vi "MyInterfaceMethod.vi"(0 "reference in":refnum<class "MyClass2.lvclass">, 1 "MyParameter":dbl, 5 "error in (no error)":errorcluster) -> (14 "reference out":refnum<class "MyClass2.lvclass">, 19 "error out":errorcluster)   [LabVIEW 2017, in "MyClass2.lvclass"]
uses:
  MyClass2.lvclass
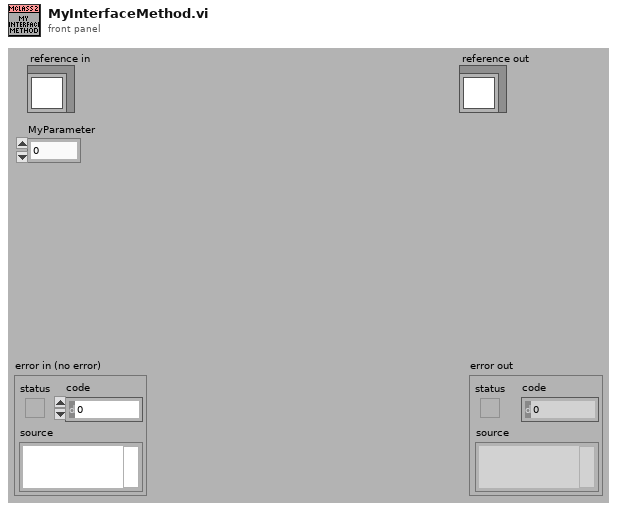
[diagram p1: front panel]
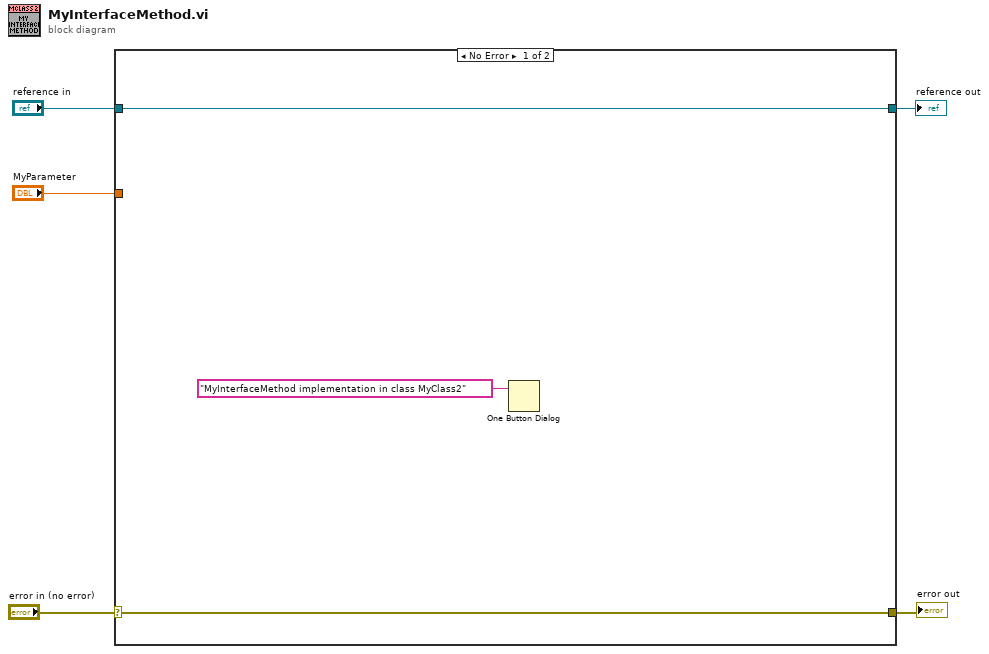
[diagram p0: block diagram]
diagram:
  n1 = case shown="No Error" "error in (no error)" {
    selector: "error in (no error)" -> [w7 w10]
    tunnel: [w7 w10] -> w4
    tunnel: [w8 w9] -> w2
    tunnel: "reference in" -> [w8 w9]
    tunnel: "MyParameter" -> [_ _]
    frame No Error {
      n2 = One Button Dialog(message="MyInterfaceMethod implementation in class MyClass2") -> ()  [unwired: 1 in, 1 out]
    }
    frame Error {
    }
  }
  "error out" <- w4
  "reference out" <- w2
